vi "Control Panel.vi"(8 "error in (no error)":errorcluster, 11 "Power Supply.lvclass":refnum<class "Power Supply.lvclass">) -> (0 "error out":errorcluster, 3 "Power Supply.lvclass out":refnum<class "Power Supply.lvclass">)   [LabVIEW 2009, in "Power Supply.lvclass"]
uses:
  Power Supply.lvclass
  Utility Classes/InstrPtr/InstrPtr.lvclass
  Magnet status.ctl
  Power Supply.lvclass/Power Supply.ctl
  File IO/File IO.lvclass
panel:
  out "Current Field":dbl[unit]
  out "Update UI":bool
  out "Status":T1
  out "*ips120":T2
  in  "Abort Field Sweep":bool
  out "done?":bool
  out "ILM Shut Down?":bool
  out "SH On":bool caption="Switch Heater"
  out "Persistent Mode":bool
  in  "SHcontrol":bool caption="Switch Heater"
  in  "gotopersistent":bool
  out "active":bool
  in  "Train\nMagnet":bool
  out "Busy":bool
  out "ready?":bool
  in  "rate":dbl[unit]=0.016666666666666666 caption="Rate" min=0.0 max=0.25
  in  "Goto":dbl[unit]
  in  "Clamp":bool
  in  "Check for Magnet":bool
  in  "Hold":bool
  in  "Goto Zero":bool
  in  "Goto Field":bool
  in  "endprgm":bool
  # "Magnet Control Panel"
  # "(at current field)"
  # "Off"
  # "On"
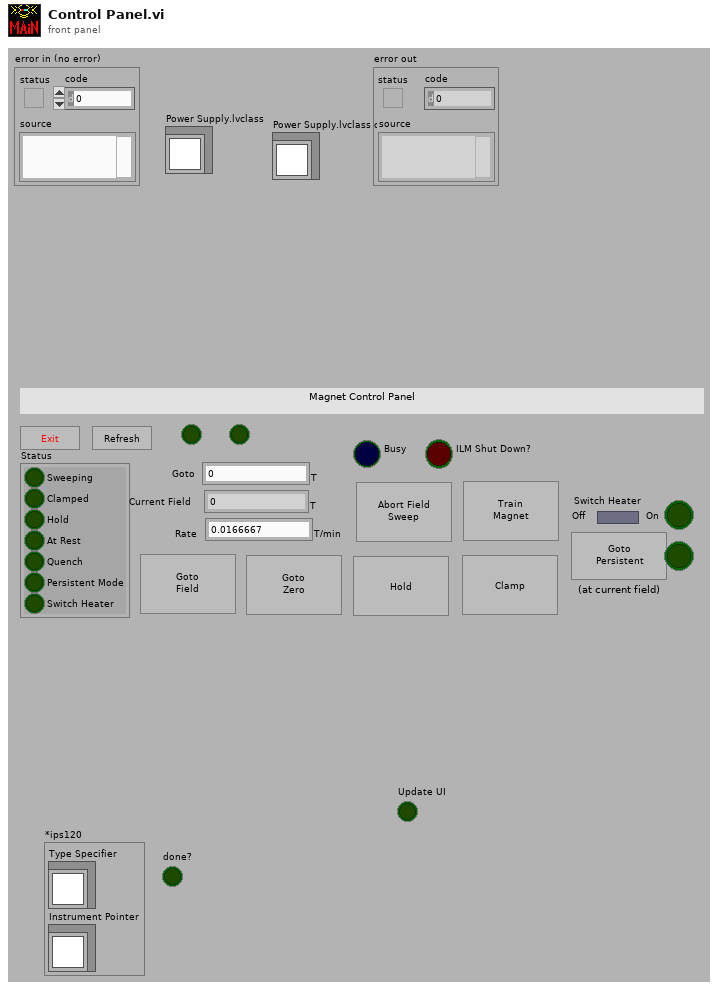
[diagram p1: front panel]
types:
  T1 = typedef "Power Supply.lvclass/Magnet status.ctl" = cluster{"Sweeping":bool, "Clamped":bool, "Hold":bool, "At Rest":bool, "Quench":bool, "Persistent Mode":bool, "Switch Heater":bool}
  T2 = cluster{"Type Specifier":refnum<class "Power Supply.lvclass">, "Instrument Pointer":refnum<class "InstrPtr.lvclass">}
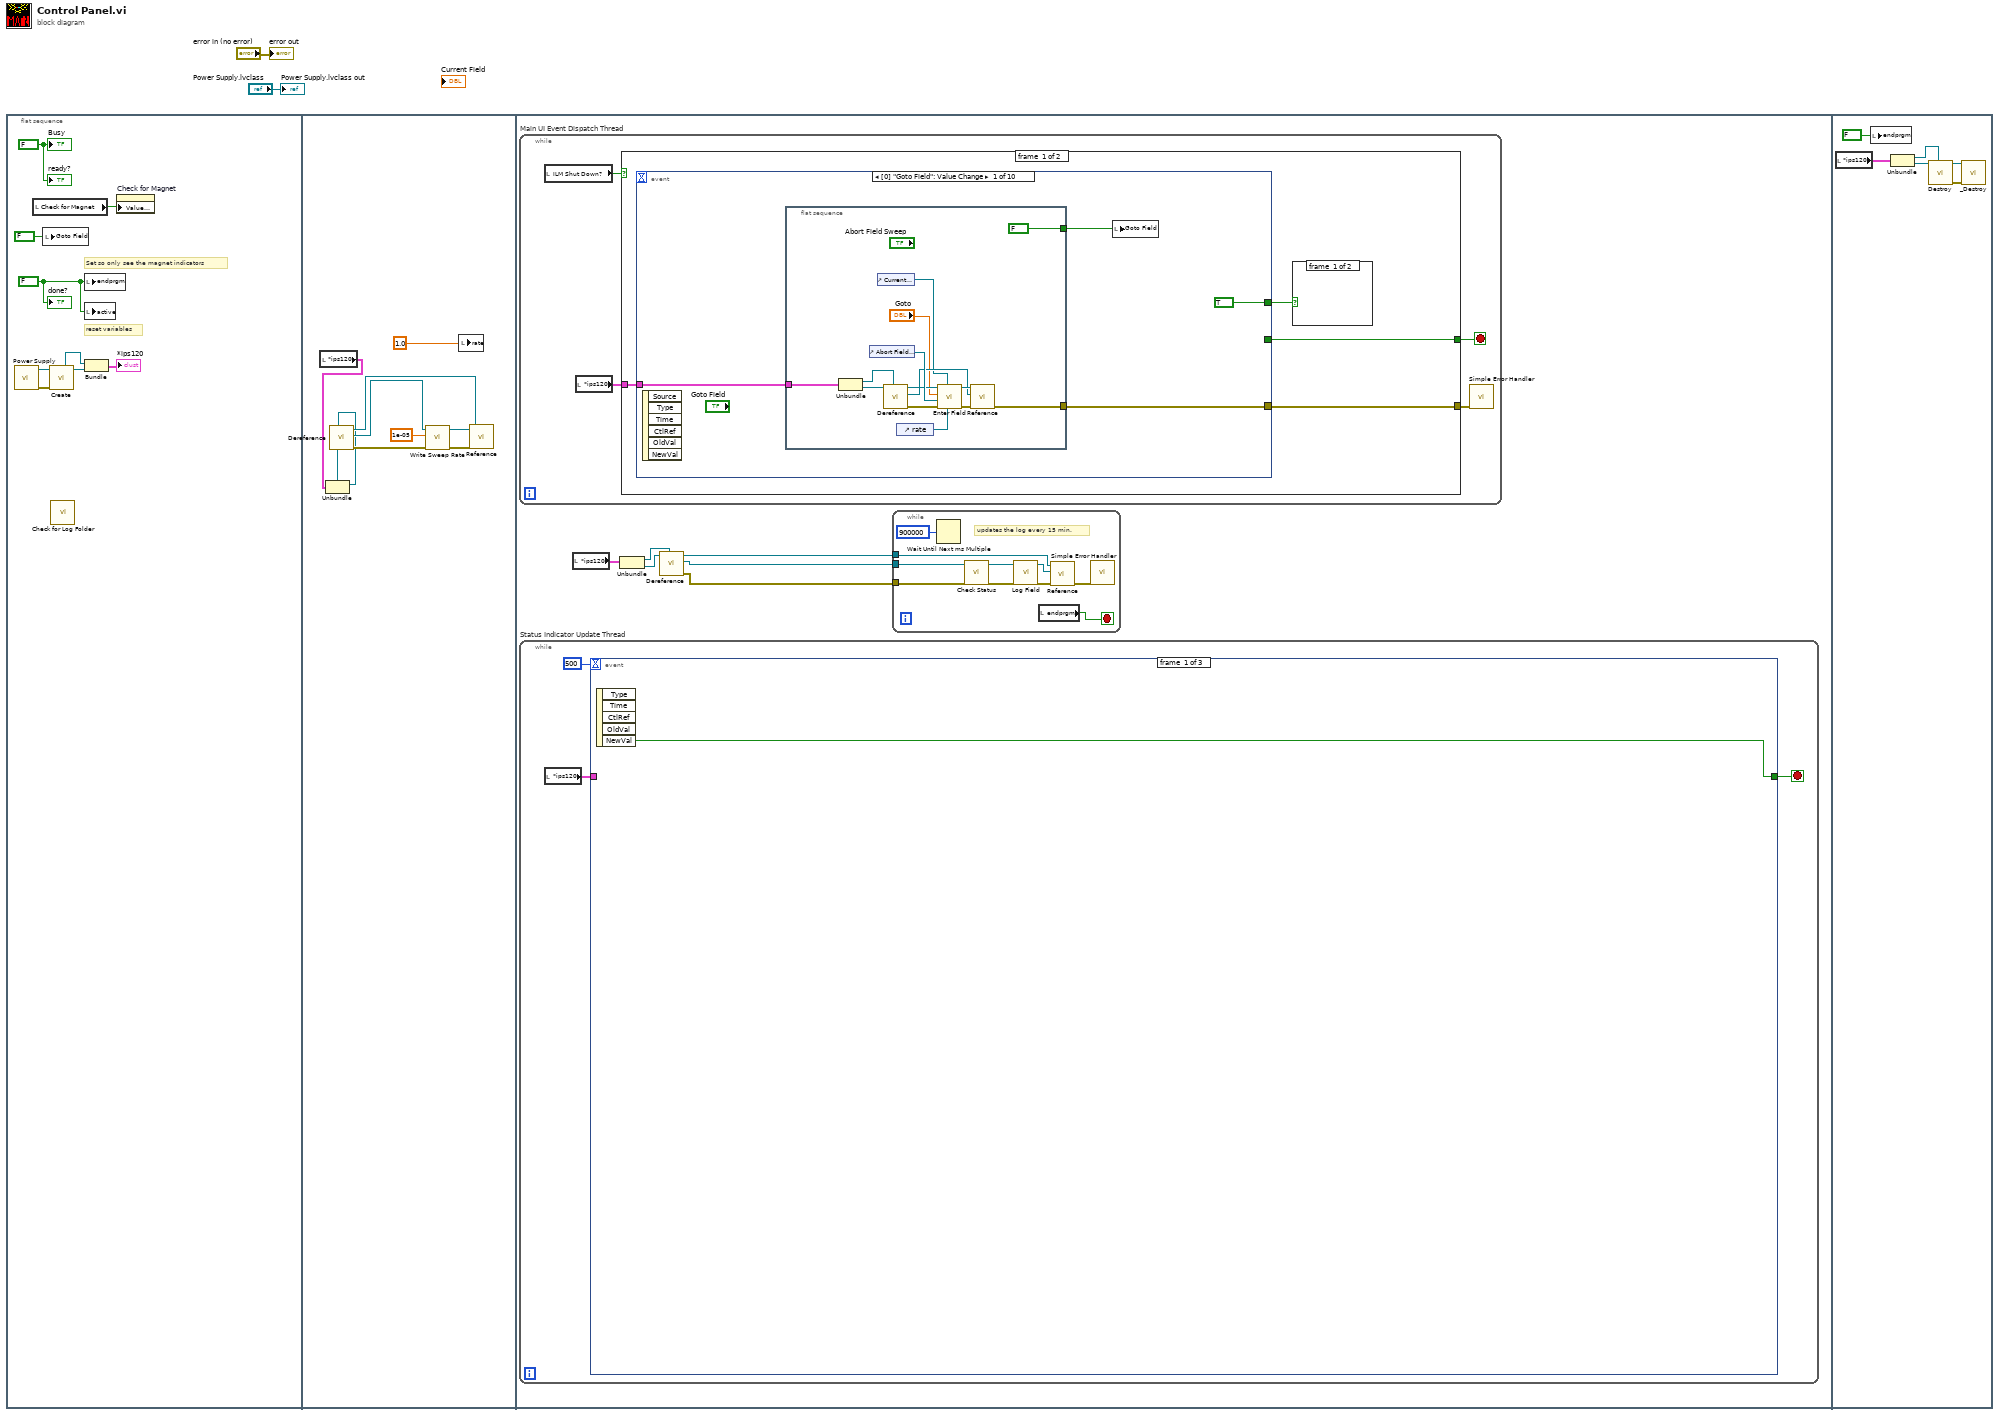
[diagram p0: block diagram]
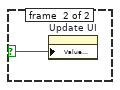
[diagram p2: hidden frame]
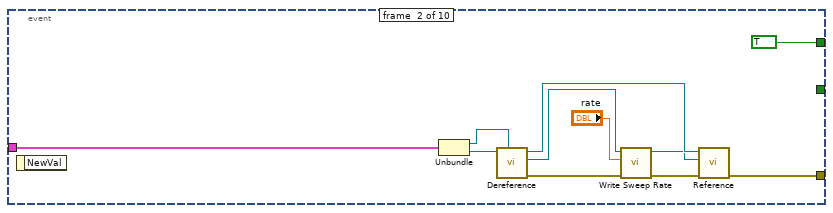
[diagram p3: hidden frame]
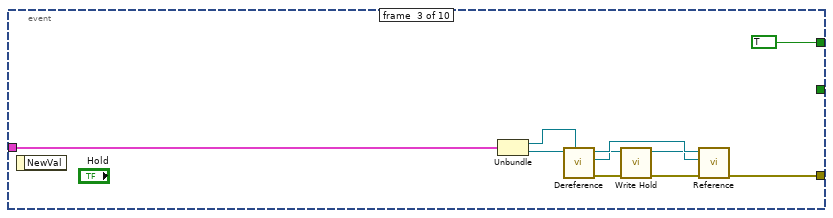
[diagram p4: hidden frame]
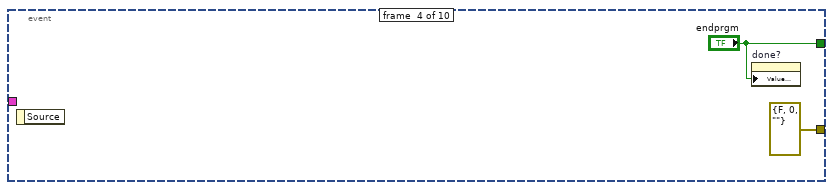
[diagram p5: hidden frame]
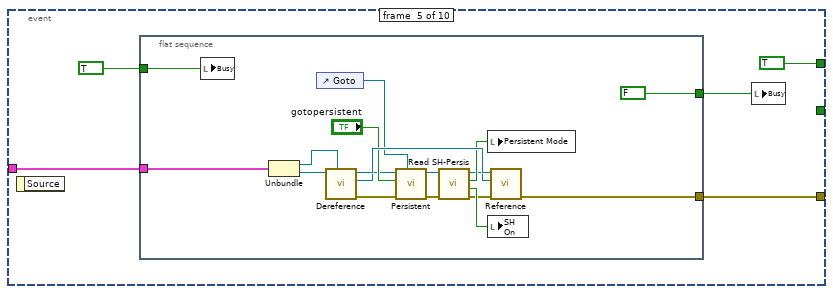
[diagram p6: hidden frame]
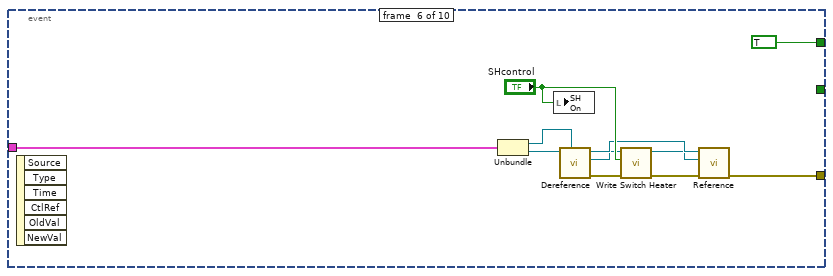
[diagram p7: hidden frame]
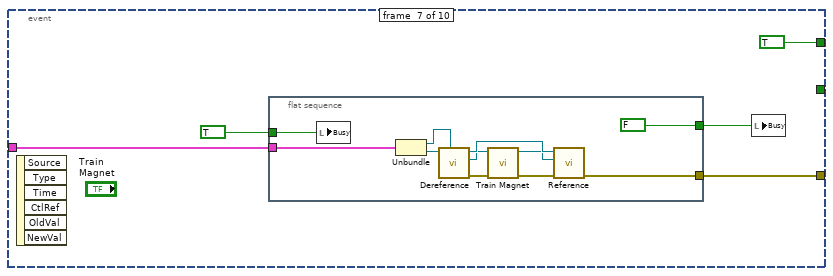
[diagram p8: hidden frame]
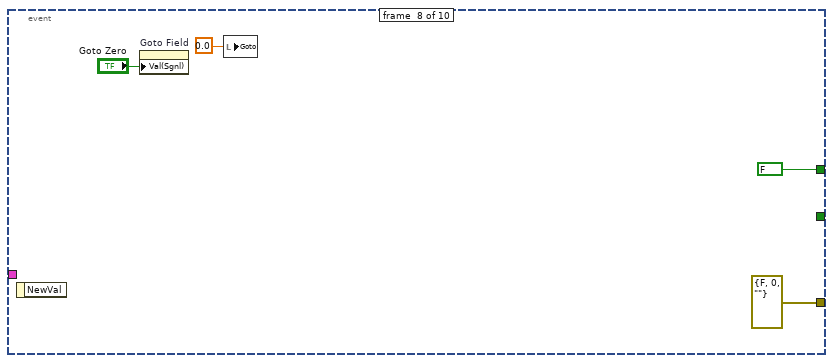
[diagram p9: hidden frame]
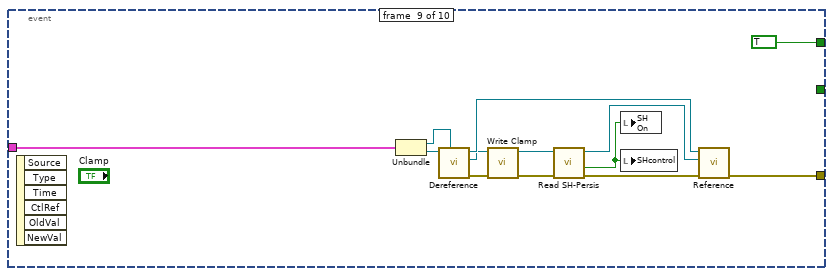
[diagram p10: hidden frame]
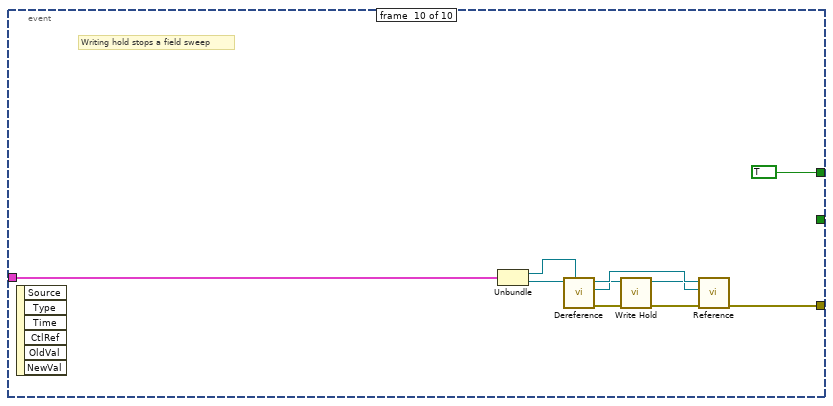
[diagram p11: hidden frame]
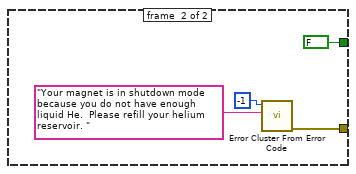
[diagram p12: hidden frame]
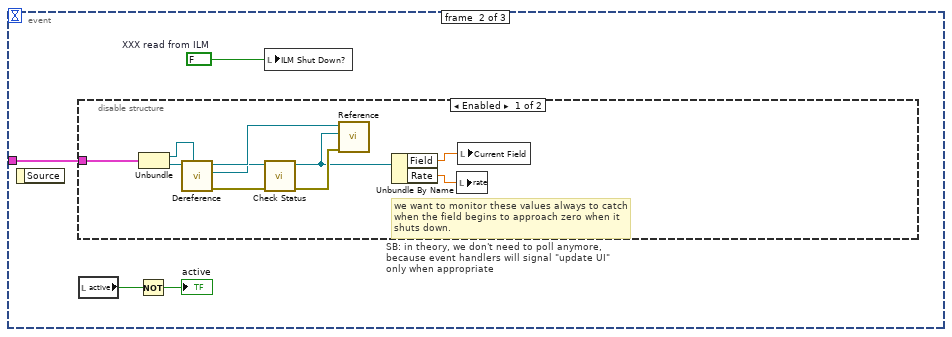
[diagram p13: hidden frame]
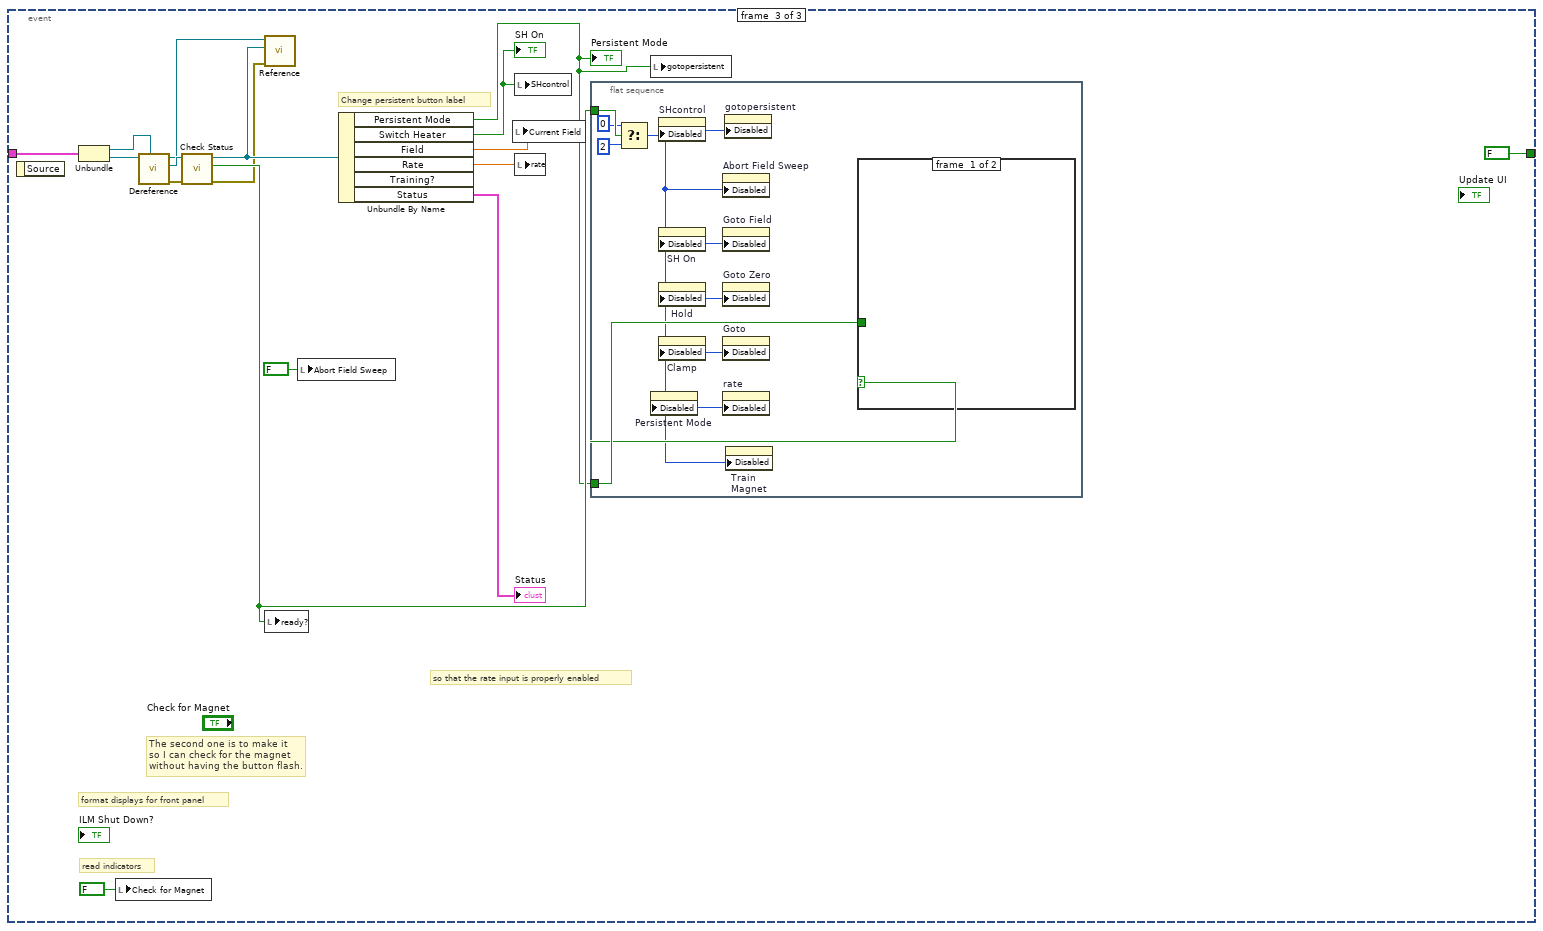
[diagram p15: hidden frame]
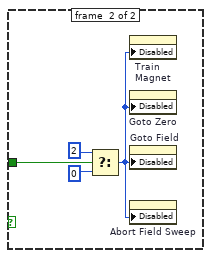
[diagram p16: hidden frame]
diagram:
  n1 = flat-sequence {
    frame #0 {
      w11 = FALSE
      w9 = FALSE
      # "Set so only see the magnet indicators"
      # "reset variables"
      n2 = call "Power Supply.vi"() -> ("error out"=w4:errorcluster, "Power Supply out"=w8:refnum<class "Power Supply.lvclass">)  [unwired: 10 in]
      n3 = local read "Check for Magnet"() -> (w10:bool)
      n4 = local write "Goto Field"(FALSE ("active")) -> ()
      n5 = call "Create.vi"("error in (no error)"=w4, "Instrument in"=w8) -> ("Instrument Pointer"=w7:refnum<class "InstrPtr.lvclass">, "Type Specifier"=w6:refnum<class "Power Supply.lvclass">)  [unwired: 7 in, 1 out]
      n6 = call "Check for Log Folder.vi"() -> ()  [unwired: 1 out]
      n7 = local write "endprgm"(w9) -> ()
      n8 = local write "active"(w9) -> ()
      n9 = Bundle("Type Specifier"=w6, "Instrument Pointer"=w7) -> (→"*ips120":T2)  [unwired: 1 in]
      n10 = property on="Check for Magnet" class="Bool (strict)"("Value (Signaling)"=w10) -> ()  [unwired: 2 in, 2 out]
      "ready?" <- w11
      "Busy" <- w11
      "done?" <- w9
    }
    frame #1 {
      n11 = local read "*ips120"() -> (w14:T2)
      n12 = Unbundle(w14) -> ("Type Specifier"=w15:refnum<class "Power Supply.lvclass">, "Instrument Pointer"=w16:refnum<class "InstrPtr.lvclass">)
      n13 = call "Dereference.vi"("Type Specifier"=w15, "InstrPtr"=w16) -> ("error out"=w20:errorcluster, "Instrument out"=w19:refnum<class "Power Supply.lvclass">, "InstrPtr out"=w17:refnum<class "InstrPtr.lvclass">)  [unwired: 7 in]
      n14 = call-dynamic "Write Sweep Rate.vi"("error in (no error)"=w20, "rate"=dbl[unit] 1e-05, "Power Supply in"=w19) -> ("error out"=w21:errorcluster, "Power Supply out"=w18:refnum<class "Power Supply.lvclass">)  [unwired: 7 in]
      n15 = local write "rate"(dbl[unit] 1.0 ("rate")) -> ()
      n16 = call "Reference.vi"("error in (no error)"=w21, "Instrument"=w18, "InstrPtr in"=w17) -> ()  [unwired: 8 in, 1 out]
    }
    frame #2 {
      n17 = while "Main UI Event Dispatch Thread" {
        stop <- w41 stop-if-true
        n18 = local read "ILM Shut Down?"() -> (w38:bool)
        n19 = local read "*ips120"() -> (w40:T2)
        n20 = case shown="False" w38 {
          tunnel: [w45 FALSE ("endprgm")] -> w41
          tunnel: w40 -> [w44 _]
          tunnel: [w43 w165] -> w39
          frame #0 {
            n21 = event shown="[0] \"Goto Field\": Value Change" {
              selector: _ -> [_ _ _ _ _ _ _ _ _ _]
              dyn-events: _ -> [_ _ _ _ _ _ _ _ _ _]
              timeout: _ -> [_ _ _ _ _ _ _ _ _ _]
              tunnel: [_ _ _ "endprgm" _ _ _ _ _ _] -> w45
              tunnel: w44 -> [w50 w75 w85 _ w92 w119 w125 _ w146 w155]
              tunnel: [w48 w66 w84 errorcluster {"status"=FALSE, "code"=0, "source"=""} ("error out") w91 w113 w124 errorcluster {"status"=FALSE, "code"=0, "source"=""} ("error out") w142 w156] -> w43
              tunnel: [TRUE TRUE TRUE _ TRUE TRUE TRUE FALSE TRUE TRUE] -> w42
              event #0 {
                n22 = event-data() -> ()  [unwired: 7 out]
                n23 = flat-sequence {
                  tunnel: w50 -> [w61]
                  tunnel: [FALSE ("Goto Field")] -> w49
                  tunnel: [w54] -> w48
                  frame #0 {
                    n24 = Unbundle(w61) -> ("Type Specifier"=w63:refnum<class "Power Supply.lvclass">, "Instrument Pointer"=w62:refnum<class "InstrPtr.lvclass">)
                    n25 = control-ref of="Abort Field Sweep"() -> (w64:refnum<vi>)
                    n26 = control-ref of="Current Field"() -> (w53:refnum<vi>)
                    n27 = call "Dereference.vi"("Type Specifier"=w63, "InstrPtr"=w62) -> ("error out"=w56:errorcluster, "Instrument out"=w60:refnum<class "Power Supply.lvclass">, "InstrPtr out"=w59:refnum<class "InstrPtr.lvclass">)  [unwired: 7 in]
                    n28 = control-ref of="rate"() -> (w51:refnum<vi>)
                    n29 = call-dynamic "Enter Field.vi"("rate monitor"=w51, "Field monitor"=w53, "error in (no error)"=w56, "Abort button"=w64, "Target field"="Goto", "Power Supply in"=w60) -> ("error out"=w57:errorcluster, "Power Supply out"=w58:refnum<class "Power Supply.lvclass">)  [unwired: 4 in]
                    n30 = call "Reference.vi"("error in (no error)"=w57, "Instrument"=w58, "InstrPtr in"=w59) -> ("error out"=w54:errorcluster)  [unwired: 8 in]
                  }
                }
                n31 = local write "Goto Field"(w49) -> ()
              }
              event #1 {
                n32 = event-data() -> ()  [unwired: 2 out]
                n33 = Unbundle(w75) -> ("Type Specifier"=w74:refnum<class "Power Supply.lvclass">, "Instrument Pointer"=w73:refnum<class "InstrPtr.lvclass">)
                n34 = call "Dereference.vi"("Type Specifier"=w74, "InstrPtr"=w73) -> ("error out"=w68:errorcluster, "Instrument out"=w70:refnum<class "Power Supply.lvclass">, "InstrPtr out"=w72:refnum<class "InstrPtr.lvclass">)  [unwired: 7 in]
                n35 = call-dynamic "Write Sweep Rate.vi"("error in (no error)"=w68, "rate"="rate", "Power Supply in"=w70) -> ("error out"=w67:errorcluster, "Power Supply out"=w71:refnum<class "Power Supply.lvclass">)  [unwired: 7 in]
                n36 = call "Reference.vi"("error in (no error)"=w67, "Instrument"=w71, "InstrPtr in"=w72) -> ("error out"=w66:errorcluster)  [unwired: 8 in]
              }
              event #2 {
                n37 = event-data() -> ()  [unwired: 2 out]
                n38 = Unbundle(w85) -> ("Type Specifier"=w82:refnum<class "Power Supply.lvclass">, "Instrument Pointer"=w83:refnum<class "InstrPtr.lvclass">)
                n39 = call "Dereference.vi"("Type Specifier"=w82, "InstrPtr"=w83) -> ("error out"=w77:errorcluster, "Instrument out"=w80:refnum<class "Power Supply.lvclass">, "InstrPtr out"=w81:refnum<class "InstrPtr.lvclass">)  [unwired: 7 in]
                n40 = call-dynamic "Write Hold.vi"("error in (no error)"=w77, "Power Supply in"=w80) -> ("error out"=w78:errorcluster, "Power Supply out"=w79:refnum<class "Power Supply.lvclass">)  [unwired: 8 in]
                n41 = call "Reference.vi"("error in (no error)"=w78, "Instrument"=w79, "InstrPtr in"=w81) -> ("error out"=w84:errorcluster)  [unwired: 8 in]
              }
              event #3 {
                n42 = event-data() -> ()  [unwired: 2 out]
                n43 = property on="done?" class="Boolean (strict)"("Value (Signaling)"="endprgm") -> ()  [unwired: 2 in, 2 out]
              }
              event #4 {
                n44 = event-data() -> ()  [unwired: 2 out]
                n45 = flat-sequence {
                  tunnel: w92 -> [w109]
                  tunnel: [w108] -> w91
                  tunnel: TRUE -> [w94]
                  tunnel: [FALSE] -> w88
                  frame #0 {
                    n46 = local write "Busy"(w94) -> ()
                    n47 = Unbundle(w109) -> ("Type Specifier"=w102:refnum<class "Power Supply.lvclass">, "Instrument Pointer"=w101:refnum<class "InstrPtr.lvclass">)
                    n48 = control-ref of="Goto"() -> (w104:refnum<vi>)
                    n49 = call "Dereference.vi"("Type Specifier"=w102, "InstrPtr"=w101) -> ("error out"=w99:errorcluster, "Instrument out"=w100:refnum<class "Power Supply.lvclass">, "InstrPtr out"=w105:refnum<class "InstrPtr.lvclass">)  [unwired: 7 in]
                    n50 = call-dynamic "Persistent.vi"("Field monitor ref"=w104, "error in (no error)"=w99, "Go to persistent mode?"="gotopersistent", "Power Supply in"=w100) -> ("error out"=w107:errorcluster, "Power Supply out"=w106:refnum<class "Power Supply.lvclass">)  [unwired: 6 in]
                    n51 = call-dynamic "Read SH-Persis.vi"("error in (no error)"=w107, "Power Supply in"=w106) -> ("error out"=w95:errorcluster, "SHon?"=w97:bool, "pers?"=w98:bool, "Power Supply out"=w96:refnum<class "Power Supply.lvclass">)  [unwired: 4 in, 2 out]
                    n52 = local write "Persistent Mode"(w98) -> ()
                    n53 = local write "SH On"(w97) -> ()
                    n54 = call "Reference.vi"("error in (no error)"=w95, "Instrument"=w96, "InstrPtr in"=w105) -> ("error out"=w108:errorcluster)  [unwired: 8 in]
                  }
                }
                n55 = local write "Busy"(w88) -> ()
              }
              event #5 {
                n56 = event-data() -> ()  [unwired: 7 out]
                n57 = Unbundle(w119) -> ("Type Specifier"=w117:refnum<class "Power Supply.lvclass">, "Instrument Pointer"=w118:refnum<class "InstrPtr.lvclass">)
                n58 = local write "SH On"("SHcontrol") -> ()
                n59 = call "Dereference.vi"("Type Specifier"=w117, "InstrPtr"=w118) -> ("error out"=w112:errorcluster, "Instrument out"=w111:refnum<class "Power Supply.lvclass">, "InstrPtr out"=w116:refnum<class "InstrPtr.lvclass">)  [unwired: 7 in]
                n60 = call-dynamic "Write Switch Heater.vi"("error in (no error)"=w112, "Turn SH On?"="SHcontrol", "Power Supply in"=w111) -> ("error out"=w114:errorcluster, "Power Supply out"=w115:refnum<class "Power Supply.lvclass">)  [unwired: 7 in]
                n61 = call "Reference.vi"("error in (no error)"=w114, "Instrument"=w115, "InstrPtr in"=w116) -> ("error out"=w113:errorcluster)  [unwired: 8 in]
              }
              event #6 {
                n62 = event-data() -> ()  [unwired: 7 out]
                n63 = flat-sequence {
                  tunnel: w125 -> [w136]
                  tunnel: [w132] -> w124
                  tunnel: [FALSE] -> w122
                  tunnel: TRUE -> [w126]
                  frame #0 {
                    n64 = local write "Busy"(w126) -> ()
                    n65 = Unbundle(w136) -> ("Type Specifier"=w135:refnum<class "Power Supply.lvclass">, "Instrument Pointer"=w134:refnum<class "InstrPtr.lvclass">)
                    n66 = call "Dereference.vi"("Type Specifier"=w135, "InstrPtr"=w134) -> ("error out"=w130:errorcluster, "Instrument out"=w131:refnum<class "Power Supply.lvclass">, "InstrPtr out"=w133:refnum<class "InstrPtr.lvclass">)  [unwired: 7 in]
                    n67 = call-dynamic "Train Magnet.vi"("error in (no error)"=w130, "Power Supply in"=w131) -> ("error out"=w129:errorcluster, "Power Supply out"=w128:refnum<class "Power Supply.lvclass">)  [unwired: 8 in]
                    n68 = call "Reference.vi"("error in (no error)"=w129, "Instrument"=w128, "InstrPtr in"=w133) -> ("error out"=w132:errorcluster)  [unwired: 8 in]
                  }
                }
                n69 = local write "Busy"(w122) -> ()
              }
              event #7 {
                n70 = event-data() -> ()  [unwired: 2 out]
                n71 = property on="Goto Field" class="Bool (strict)"("Val(Sgnl)"="Goto Zero") -> ()  [unwired: 2 in, 2 out]
                n72 = local write "Goto"(dbl[unit] 0.0 ("Goto")) -> ()
              }
              event #8 {
                n73 = event-data() -> ()  [unwired: 7 out]
                n74 = Unbundle(w146) -> ("Type Specifier"=w150:refnum<class "Power Supply.lvclass">, "Instrument Pointer"=w149:refnum<class "InstrPtr.lvclass">)
                n75 = call "Dereference.vi"("Type Specifier"=w150, "InstrPtr"=w149) -> ("error out"=w145:errorcluster, "Instrument out"=w147:refnum<class "Power Supply.lvclass">, "InstrPtr out"=w148:refnum<class "InstrPtr.lvclass">)  [unwired: 7 in]
                n76 = call-dynamic "Write Clamp.vi"("error in (no error)"=w145, "Power Supply in"=w147) -> ("error out"=w152:errorcluster, "Power Supply out"=w153:refnum<class "Power Supply.lvclass">)  [unwired: 8 in]
                n77 = call-dynamic "Read SH-Persis.vi"("error in (no error)"=w152, "Power Supply in"=w153) -> ("error out"=w144:errorcluster, "SHon?"=w151:bool, "Power Supply out"=w143:refnum<class "Power Supply.lvclass">)  [unwired: 4 in, 3 out]
                n78 = local write "SH On"(w151) -> ()
                n79 = local write "SHcontrol"(w151) -> ()
                n80 = call "Reference.vi"("error in (no error)"=w144, "Instrument"=w143, "InstrPtr in"=w148) -> ("error out"=w142:errorcluster)  [unwired: 8 in]
              }
              event #9 {
                # "Writing hold stops a field sweep"
                n81 = event-data() -> ()  [unwired: 7 out]
                n82 = Unbundle(w155) -> ("Type Specifier"=w163:refnum<class "Power Supply.lvclass">, "Instrument Pointer"=w162:refnum<class "InstrPtr.lvclass">)
                n83 = call "Dereference.vi"("Type Specifier"=w163, "InstrPtr"=w162) -> ("error out"=w160:errorcluster, "Instrument out"=w157:refnum<class "Power Supply.lvclass">, "InstrPtr out"=w161:refnum<class "InstrPtr.lvclass">)  [unwired: 7 in]
                n84 = call-dynamic "Write Hold.vi"("error in (no error)"=w160, "Power Supply in"=w157) -> ("error out"=w159:errorcluster, "Power Supply out"=w158:refnum<class "Power Supply.lvclass">)  [unwired: 8 in]
                n85 = call "Reference.vi"("error in (no error)"=w159, "Instrument"=w158, "InstrPtr in"=w161) -> ("error out"=w156:errorcluster)  [unwired: 8 in]
              }
            }
            n86 = case shown="True" w42 {
              selector: w42 -> [_ w46]
              frame #0 {
              }
              frame #1 {
                n87 = property on="Update UI" class="Bool (strict)"("Value (Signaling)"=w46) -> ()  [unwired: 2 in, 2 out]
              }
            }
          }
          frame #1 {
            n88 = call <vilib>:"Error Cluster From Error Code.vi"("error message (\"\")"="Your magnet is in shutdown mode because you do not have enough liquid He.  Please refill your helium reservoir. ", "error code (0)"=-1) -> ("error out"=w165:errorcluster)  [unwired: 7 in]
          }
        }
        n89 = call <vilib>:"Simple Error Handler.vi"("error in (no error)"=w39) -> ()  [unwired: 4 in, 5 out]
      }
      n90 = while "Status Indicator Update Thread" {
        stop <- w169 stop-if-true
        n91 = local read "*ips120"() -> (w168:T2)
        n92 = event shown="[1] Timeout" {
          selector: _ -> [_ _ _]
          dyn-events: _ -> [_ _ _]
          timeout: 500 -> [_ _ _]
          tunnel: [w171 _ FALSE] -> w169
          tunnel: w168 -> [_ w173 w192]
          event #0 {
            n93 = event-data() -> ("NewVal"=w171:bool)  [unwired: 5 out]
          }
          event #1 {
            w172 = FALSE  # XXX read from ILM
            n94 = event-data() -> ()  [unwired: 2 out]
            n95 = disable-structure "SB: in theory, we don't need to poll anymore, because event handlers will signal \"update UI\" only when appropriate" shown="Enabled" {
              disable-tunnel: w173 -> [w181 _]
              frame #0 {
                # "we want to monitor these values always to catch\nwhen the field begins to approach zero when it\nshuts down."
                n96 = Unbundle(w181) -> ("Type Specifier"=w183:refnum<class "Power Supply.lvclass">, "Instrument Pointer"=w184:refnum<class "InstrPtr.lvclass">)
                n97 = call "Dereference.vi"("Type Specifier"=w183, "InstrPtr"=w184) -> ("error out"=w180:errorcluster, "Instrument out"=w179:refnum<class "Power Supply.lvclass">, "InstrPtr out"=w185:refnum<class "InstrPtr.lvclass">)  [unwired: 7 in]
                n98 = call-dynamic "Check Status.vi"("error in (no error)"=w180, "Power Supply in"=w179) -> ("error out"=w182:errorcluster, "Power Supply out"=w178:refnum<class "Power Supply.lvclass">)  [unwired: 6 in, 2 out]
                n99 = call "Reference.vi"("error in (no error)"=w182, "Instrument"=w178, "InstrPtr in"=w185) -> ()  [unwired: 8 in, 1 out]
                n100 = Unbundle By Name(w178) -> ("Field"=w176:dbl[unit], "Rate"=w177:dbl[unit])
                n101 = local write "rate"(w177) -> ()
                n102 = local write "Current Field"(w176) -> ()
              }
              frame #1 {
              }
            }
            n103 = local read "active"() -> (w175:bool)
            n104 = Not(x=w175) -> (.not. x?=→"active":bool)
            n105 = local write "ILM Shut Down?"(w172) -> ()
          }
          event #2 {
            # "format displays for front panel"
            # "read indicators"
            # "so that the rate input is properly enabled"
            # "Change persistent button label"
            # "The second one is to make it\nso I can check for the magnet\nwithout having the button flash."
            n106 = event-data() -> ()  [unwired: 2 out]
            n107 = Unbundle(w192) -> ("Type Specifier"=w193:refnum<class "Power Supply.lvclass">, "Instrument Pointer"=w198:refnum<class "InstrPtr.lvclass">)
            n108 = local write "Check for Magnet"(FALSE) -> ()
            n109 = call "Dereference.vi"("Type Specifier"=w193, "InstrPtr"=w198) -> ("error out"=w197:errorcluster, "Instrument out"=w196:refnum<class "Power Supply.lvclass">, "InstrPtr out"=w194:refnum<class "InstrPtr.lvclass">)  [unwired: 7 in]
            n110 = call-dynamic "Check Status.vi"("error in (no error)"=w197, "Power Supply in"=w196) -> ("error out"=w191:errorcluster, "Ready?"=w200:bool, "Power Supply out"=w195:refnum<class "Power Supply.lvclass">)  [unwired: 6 in, 1 out]
            n111 = call "Reference.vi"("error in (no error)"=w191, "Instrument"=w195, "InstrPtr in"=w194) -> ()  [unwired: 8 in, 1 out]
            n112 = local write "ready?"(w200) -> ()
            n113 = local write "Abort Field Sweep"(FALSE ("Abort Field Sweep")) -> ()
            n114 = Unbundle By Name(w195) -> ("Persistent Mode"=w187:bool, "Switch Heater"=w199:bool, "Field"=w188:dbl[unit], "Rate"=w189:dbl[unit], "Status"=→"Status":T1)  [unwired: 1 out]
            "Persistent Mode" <- w187
            "SH On" <- w199
            n115 = local write "Current Field"(w188) -> ()
            n116 = local write "SHcontrol"(w199) -> ()
            n117 = local write "rate"(w189) -> ()
            n118 = flat-sequence {
              tunnel: w187 -> [w207]
              tunnel: w200 -> [w206]
              frame #0 {
                n119 = Select(t=0, s=w206, f=2) -> (s? t:f=w203:i32)
                n120 = property on="Persistent Mode" class="Boolean (strict)"("Disabled"=w203) -> ()  [unwired: 2 in, 2 out]
                n121 = property on="SHcontrol" class="Boolean (strict)"("Disabled"=w203) -> ()  [unwired: 2 in, 2 out]
                n122 = property on="SH On" class="Boolean (strict)"("Disabled"=w203) -> ()  [unwired: 2 in, 2 out]
                n123 = property on="Hold" class="Boolean"("Disabled"=w203) -> ()  [unwired: 2 in, 2 out]
                n124 = property on="Clamp" class="Boolean"("Disabled"=w203) -> ()  [unwired: 2 in, 2 out]
                n125 = property on="Abort Field Sweep" class="Bool (strict)"("Disabled"=w203) -> ()  [unwired: 2 in, 2 out]
                n126 = property on="Goto Field" class="Bool (strict)"("Disabled"=w203) -> ()  [unwired: 2 in, 2 out]
                n127 = property on="Goto Zero" class="Boolean"("Disabled"=w203) -> ()  [unwired: 2 in, 2 out]
                n128 = property on="Goto" class="DigNum (strict)"("Disabled"=w203) -> ()  [unwired: 2 in, 2 out]
                n129 = property on="rate" class="DigNum (strict)"("Disabled"=w203) -> ()  [unwired: 2 in, 2 out]
                n130 = property on="gotopersistent" class="Bool (strict)"("Disabled"=w203) -> ()  [unwired: 2 in, 2 out]
                n131 = property on="Train\nMagnet" class="Boolean"("Disabled"=w203) -> ()  [unwired: 2 in, 2 out]
                n132 = case shown="True" w206 {
                  tunnel: w207 -> [_ w209]
                  frame #0 {
                  }
                  frame #1 {
                    n133 = Select(t=2, s=w209, f=0) -> (s? t:f=w208:i32)
                    n134 = property on="Train\nMagnet" class="Boolean"("Disabled"=w208) -> ()  [unwired: 2 in, 2 out]
                    n135 = property on="Goto Zero" class="Bool"("Disabled"=w208) -> ()  [unwired: 2 in, 2 out]
                    n136 = property on="Goto Field" class="Bool (strict)"("Disabled"=w208) -> ()  [unwired: 2 in, 2 out]
                    n137 = property on="Abort Field Sweep" class="Bool (strict)"("Disabled"=w208) -> ()  [unwired: 2 in, 2 out]
                  }
                }
              }
            }
            n138 = local write "gotopersistent"(w187) -> ()
          }
        }
      }
      n139 = local read "*ips120"() -> (w27:T2)
      n140 = Unbundle(w27) -> ("Type Specifier"=w26:refnum<class "Power Supply.lvclass">, "Instrument Pointer"=w25:refnum<class "InstrPtr.lvclass">)
      n141 = call "Dereference.vi"("Type Specifier"=w26, "InstrPtr"=w25) -> ("error out"=w23:errorcluster, "Instrument out"=w24:refnum<class "Power Supply.lvclass">, "InstrPtr out"=w22:refnum<class "InstrPtr.lvclass">)  [unwired: 7 in]
      n142 = while {
        tunnel: w24 -> [w34]
        tunnel: w23 -> [w33]
        tunnel: w22 -> [w29]
        stop <- w28 stop-if-true
        # "updates the log every 15 min."
        n143 = Wait Until Next ms Multiple(millisecond multiple=u32 900000) -> ()  [unwired: 1 out]
        n144 = call-dynamic "Check Status.vi"("error in (no error)"=w33, "Power Supply in"=w34) -> ("error out"=w36:errorcluster, "Power Supply out"=w35:refnum<class "Power Supply.lvclass">)  [unwired: 6 in, 2 out]
        n145 = call "Log Field.vi"("error in (no error)"=w36, "Power Supply In"=w35) -> ("error out"=w32:errorcluster, "Power Supply Out"=w31:refnum<class "Power Supply.lvclass">)  [unwired: 8 in]
        n146 = local read "endprgm"() -> (w28:bool)
        n147 = call "Reference.vi"("error in (no error)"=w32, "Instrument"=w31, "InstrPtr in"=w29) -> ("error out"=w30:errorcluster)  [unwired: 8 in]
        n148 = call <vilib>:"Simple Error Handler.vi"("error in (no error)"=w30) -> ()  [unwired: 4 in, 5 out]
      }
    }
    frame #3 {
      n149 = local read "*ips120"() -> (w216:T2)
      n150 = local write "endprgm"(FALSE) -> ()
      n151 = Unbundle(w216) -> ("Type Specifier"=w213:refnum<class "Power Supply.lvclass">, "Instrument Pointer"=w215:refnum<class "InstrPtr.lvclass">)
      n152 = call "Destroy.vi"("Type Specifier"=w213, "InstrPtr in"=w215) -> ("error out"=w212:errorcluster, "final Instrument"=w214:refnum<class "Power Supply.lvclass">)  [unwired: 8 in]
      n153 = call-dynamic "_Destroy.vi"("error in (no error)"=w212, "Instrument in"=w214) -> ()  [unwired: 9 in, 1 out]
    }
  }
  "Power Supply.lvclass out" <- "Power Supply.lvclass"
  "error out" <- "error in (no error)"
